vi "GEA2 Serial Get CRC1.vi"(8 "Error In":errorcluster, 10 "Current Read Index":i32, 11 "ReadArray":u8[](array[numeric])) -> (0 "Error Out":errorcluster, 2 "CRC Read":u8[](array[numeric]), 3 "Current Read Index":i32)   [LabVIEW 2014]
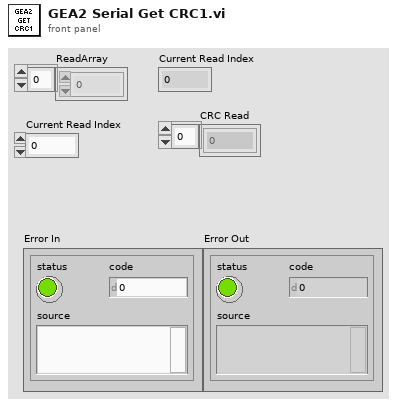
[diagram p1: front panel]
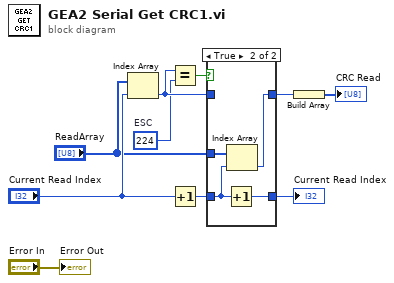
[diagram p0: block diagram]
diagram:
  w2 = u8 224  # ESC
  n1 = Index Array(array="ReadArray", index="Current Read Index") -> (element=w9:u8)
  n2 = Equal?(x=w9, y=w2) -> (x = y?=w3:bool)
  n3 = Increment(x="Current Read Index") -> (x+1=w8:i32)
  n4 = case shown="True" w3 {
    tunnel: [w11 w13] -> w5
    tunnel: [w12 w16] -> w4
    tunnel: "ReadArray" -> [_ w15]
    tunnel: w8 -> [w12 w14]
    tunnel: w9 -> [w11 _]
    frame False {
    }
    frame True {
      n5 = Increment(x=w14) -> (x+1=w16:i32)
      n6 = Index Array(array=w15, index=w14) -> (element=w13:u8)
    }
  }
  "Current Read Index" <- w4
  n7 = Build Array(w5) -> (→"CRC Read":u8[])
  "Error Out" <- "Error In"
